vi "Test Base Function.vi"(8 "error in (no error)":errorcluster, 11 "Base Class Test In":refnum<class "Base Class Test.lvclass">) -> (0 "error out":errorcluster, 3 "Base Class Test Out":refnum<class "Base Class Test.lvclass">)   [LabVIEW 2020, in "Base Class Test.lvclass"]
uses:
  Base Class Test.lvclass
  C:/Program Files (x86)/National Instruments/LabVIEW 2020/vi.lib/Asteme/LUnit/Test Case.lvclass
  Base Class Test.lvclass/Base Class Test.ctl
  <vilib>/Asteme/LUnit/Test Case.lvclass/Test Case.ctl
  <vilib>/Asteme/LUnit/LUnit Assertion Result.lvclass/LUnit Assertion Result.ctl
  <vilib>/Asteme/LUnit/Palette/Pass.vi
  <vilib>/Asteme/LUnit/Palette/Fail.vi
  <vilib>/Asteme/LUnit/Variant to string.vi
  <vilib>/Asteme/LUnit/Set Assertion Type.vi
  <vilib>/Asteme/LUnit/Add test result.vi
  <vilib>/Asteme/LUnit/LUnit Write Passed.vi
  <vilib>/Asteme/LUnit/LUnit Get Test Case.vi
  <vilib>/Asteme/LUnit/LUnit Write Message.vi
  <vilib>/Asteme/LUnit/LUnit Write Description.vi
  <vilib>/Asteme/LUnit/LUnit Write Assertion Type.vi
  <vilib>/Asteme/LUnit/Read Test Case Name.vi
  <vilib>/Asteme/LUnit/Assertion Result/LUnit Get Test Name.vi
  <vilib>/Utility/Data Type/Get Type Information.vi
  <vilib>/Utility/LVClass/Get LV Class Name.vi
  Framework/Base/Base.lvclass
  <vilib>/Asteme/LUnit/LUnit Assertion Result.lvclass
  <vilib>/Asteme/LUnit/Test Case.lvclass
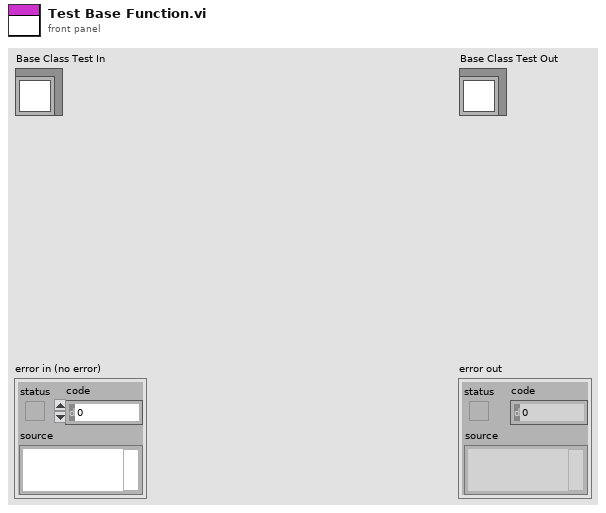
[diagram p1: front panel]
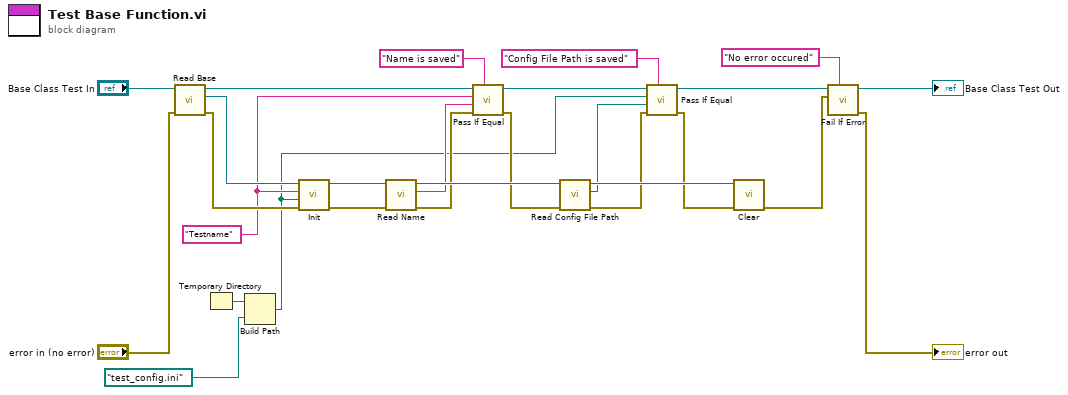
[diagram p0: block diagram]
diagram:
  w17 = "Testname" ("Name")
  n1 = call "Read Base.vi"("error in (no error)"="error in (no error)", "Base Class Test In"="Base Class Test In") -> ("error out"=w19:errorcluster, "Base.lvclass"=w21:refnum<class "Base.lvclass">, "Base Class Test Out"=w22:refnum<class "Base Class Test.lvclass">)  [unwired: 7 in]
  n2 = Temporary Directory() -> (w3:path)
  n3 = Build Path(base path=w3, name or relative path=path "test_config.ini" ("Config File Path")) -> (appended path=w2:path)
  n4 = call-dynamic "Init.vi"("error in (no error)"=w19, "Config File Path"=w2, "Name"=w17, "Base In"=w21) -> ("error out"=w25:errorcluster, "Base Out"=w26:refnum<class "Base.lvclass">)  [unwired: 6 in]
  n5 = call-dynamic "Read Name.vi"("error in (no error)"=w25, "Base In"=w26) -> ("error out"=w15:errorcluster, "Qualified Name"=w16:string, "Base Out"=w24:refnum<class "Base.lvclass">)  [unwired: 6 in, 1 out]
  n6 = call <vilib>:"Pass If Equal.vi"("Description"="Name is saved", "error in (no error)"=w15, "Actual"=w16, "Expected"=w17, "Test Case In"=w22) -> ("error out"=w14:errorcluster, "Test Case Out"=w18:refnum<class "Base Class Test.lvclass">)  [unwired: 5 in]
  n7 = call-dynamic "Read Config File Path.vi"("error in (no error)"=w14, "Process In"=w24) -> ("error out"=w12:errorcluster, "Config File Path"=w13:path, "Process Out"=w23:refnum<class "Base.lvclass">)  [unwired: 7 in]
  n8 = call <vilib>:"Pass If Equal.vi"("Description"="Config File Path is saved", "error in (no error)"=w12, "Actual"=w13, "Expected"=w2, "Test Case In"=w18) -> ("error out"=w11:errorcluster, "Test Case Out"=w8:refnum<class "Base Class Test.lvclass">)  [unwired: 5 in]
  n9 = call-dynamic "Clear.vi"("error in (no error)"=w11, "Base In"=w23) -> ("error out"=w6:errorcluster)  [unwired: 8 in, 1 out]
  n10 = call <vilib>:"Fail If Error.vi"("Description"="No error occured", "Assert error"=w6, "Test Case In"=w8) -> ("error out"=→"error out":errorcluster, "Test Case Out"=→"Base Class Test Out":refnum<class "Base Class Test.lvclass">)  [unwired: 7 in]
